vi "Test Positive Semi Definite (DBL).vi"(10 "relative tolerance":dbl=-1.0, 11 "Input Matrix":T1) -> (0 "error":i32, 3 "positive semidefinite?":bool)   [LabVIEW 2020, in "NI_AALPro.lvlib"]
uses:
  <vilib>/Analysis/NI_AALPro.lvlib
  <vilib>/Analysis/Matrix/Datatypes/RealMatrix.ctl
  <resource>/lvanlys.dll
  <vilib>/Analysis/Matrix/NI_Matrix.lvlib
panel:
  # "Test Positive Semi Definite"
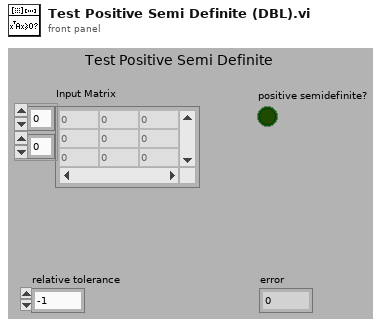
[diagram p1: front panel]
types:
  T1 = typedef "NI_Matrix.lvlib/RealMatrix.ctl" = dbl[][]
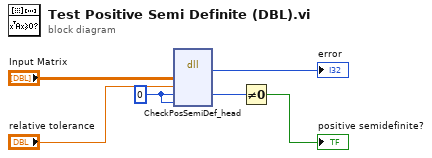
[diagram p0: block diagram]
diagram:
  w2 = 0 ("_possemidef")
  n1 = dll-call lib="e:/builds/penguin/labview/branches/2020/dev/dist/resource/lvanlys.*" fn="CheckPosSemiDef_head"("_aH"="Input Matrix", "_tol"="relative tolerance", "_possemidef"=w2, "_rank"=w2) -> ("return type"=→"error":i32, "_possemidef"=w1:i32)  [unwired: 6 in, 2 out]
  n2 = Not Equal To 0?(x=w1) -> (x != 0?=→"positive semidefinite?":bool)
